vi "Main.vi"(0 "A":dbl=4.0 min=0.0, 5 "B":dbl=2.0, 7 "Calculate":bool, 11 "error in (no error)":errorcluster, 13 "Operation":T1) -> (4 "C":dbl=6.0, 15 "error out":errorcluster)   [LabVIEW 2021, in "Calculator.lvlib"]
doc: "This VI acts as a simple calculator using OOPS . There are four seperate child classes for each arithmetic operation which has its overriding method operation.vi . The user selects the operation to perform and gives the input. The output is displayed when calculate is pressed."
uses:
  Calculator.lvlib
  Controls/QueueOperations.ctl
  Controls/Operation.ctl
  Controls/DataCluster.ctl
  Classes/NumericOperation/NumericOperation.lvclass
  Classes/Child/Add/Add.lvclass
  Classes/Child/Subtract/Subtract.lvclass
  Classes/Child/Multiply/Multiply.lvclass
  Classes/Child/Divide/Divide.lvclass
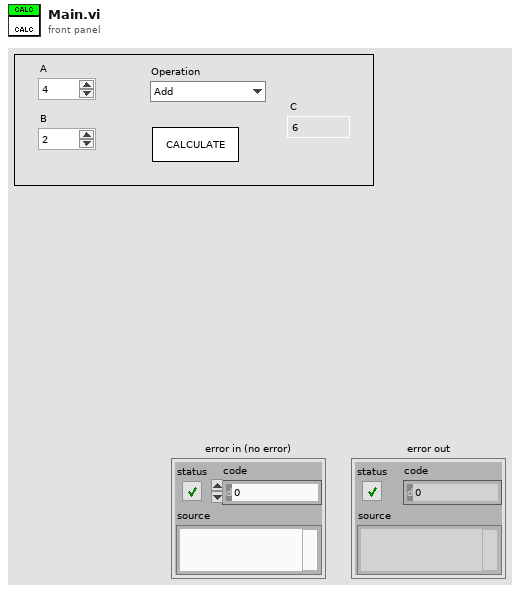
[diagram p1: front panel]
types:
  T1 = typedef "Calculator.lvlib/Operation.ctl" = enum16{"Add", "Subtract", "Multiply", "Divide"}
  T2 = typedef "Calculator.lvlib/QueueOperations.ctl" = enum16{"Create", "Enqueue", "EnqueueN", "Enqueue at Top", "Dequeue", "Flush", "Release"}
  T3 = typedef "Calculator.lvlib/DataCluster.ctl" = cluster{"A":dbl, "B":dbl, "C":dbl, "Operation":T1, "NumericOperation.lvclass":refnum<class "NumericOperation.lvclass">, "generic class reference":refnum<class "NumericOperation.lvclass">}
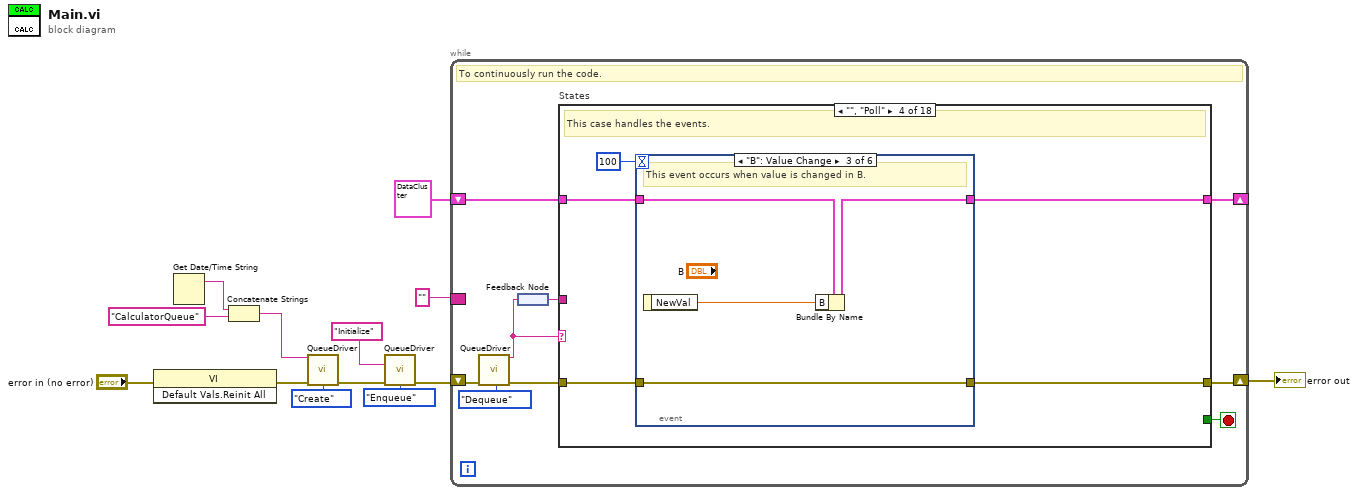
[diagram p0: block diagram]
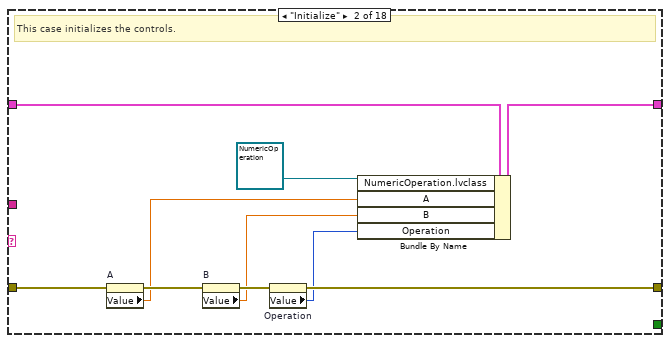
[diagram p3: hidden frame]
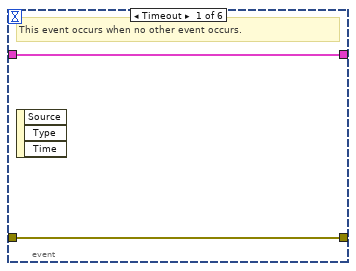
[diagram p5: hidden frame]
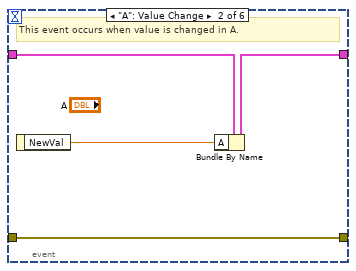
[diagram p6: hidden frame]
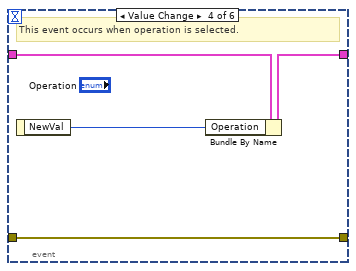
[diagram p7: hidden frame]
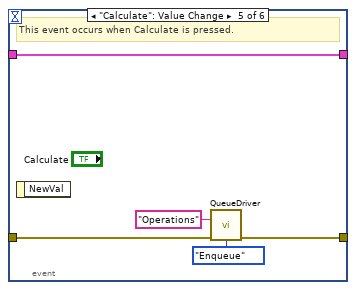
[diagram p8: hidden frame]
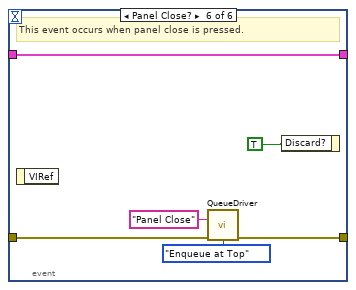
[diagram p9: hidden frame]
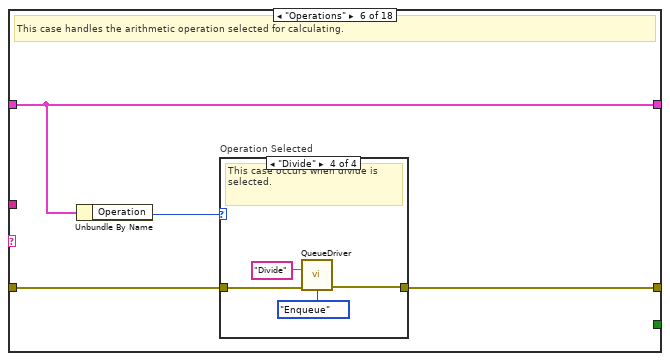
[diagram p11: hidden frame]
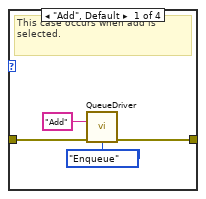
[diagram p12: hidden frame]
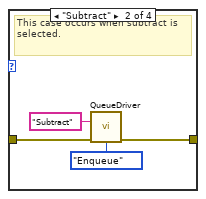
[diagram p13: hidden frame]
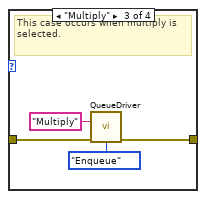
[diagram p14: hidden frame]
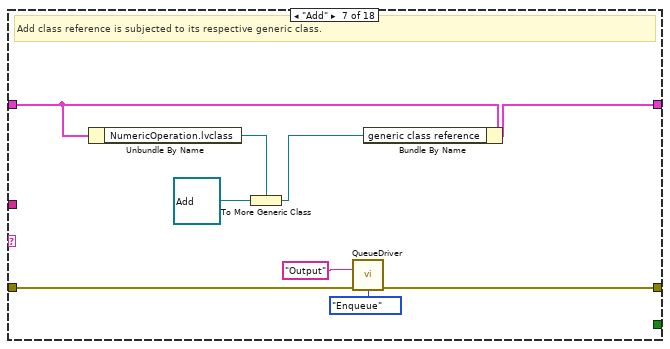
[diagram p15: hidden frame]
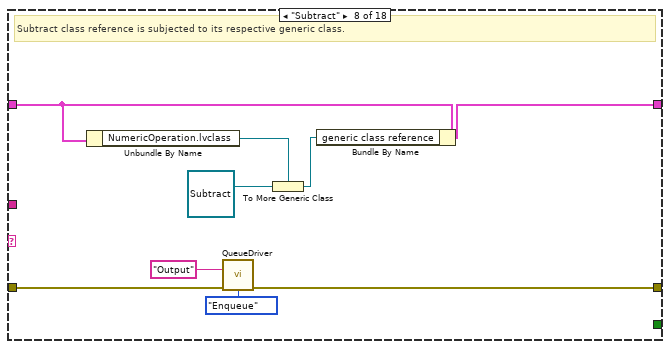
[diagram p16: hidden frame]
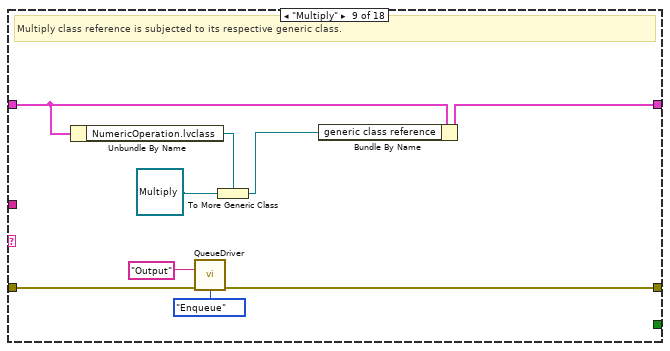
[diagram p17: hidden frame]
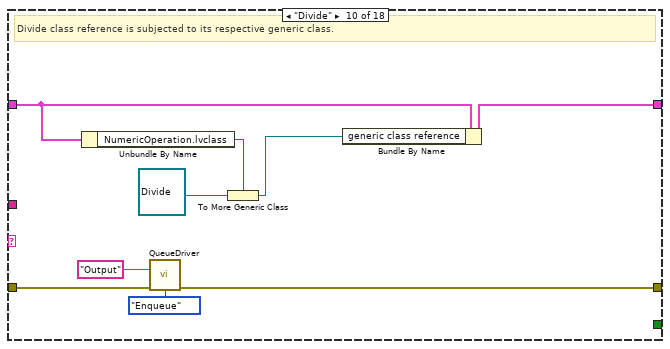
[diagram p18: hidden frame]
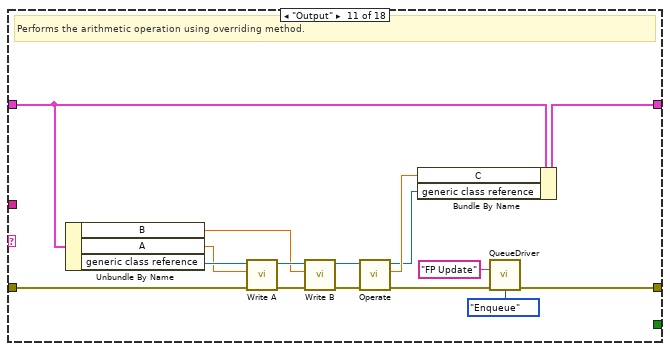
[diagram p19: hidden frame]
diagram:
  n1 = invoke class="VI" method="Default Vals.Reinit All"(error in="error in (no error)") -> (error out=w1:errorcluster)  [unwired: 2 in, 2 out]
  n2 = Get Date/Time String() -> (date string=w5:string)  [unwired: 3 in, 1 out]
  n3 = Concatenate Strings(w5, "CalculatorQueue" ("Queue Name")) -> (w3:string)
  n4 = call "QueueDriver.vi"("Queue Name"=w3, "error in (no error)"=w1, "Queue Operations"=QueueOperations."Create") -> ("error out"=w10:errorcluster)  [unwired: 11 in, 1 out]
  n5 = call "QueueDriver.vi"("State"="Initialize", "error in (no error)"=w10, "Queue Operations"=QueueOperations."Enqueue") -> ("error out"=w7:errorcluster)  [unwired: 11 in, 1 out]
  n6 = while {
    shift-right: [w20] -> _
    shift-left: T3 {"A"=0.0, "B"=0.0, "C"=0.0, "Operation"=enum."Add", "NumericOperation.lvclass"=refnum, "generic class reference"=refnum} -> [w21]
    shift-right: [w18] -> w12
    shift-left: w7 -> [w19]
    border: "" ("Dequeued Element") -> [_]
    stop <- w15 stop-if-true
    # "To continuously run the code."
    n7 = call "QueueDriver.vi"("error in (no error)"=w19, "Queue Operations"=QueueOperations."Dequeue") -> ("Dequeued Element"=w17:string, "error out"=w14:errorcluster)  [unwired: 12 in]
    n8 = feedback-in #1(w17) -> ()
    n9 = feedback #1() -> (w16:string)
    n10 = case "States" shown="\"\", \"Poll\"" w17 {
      tunnel: w21 -> [w24 w34 w36 w40 w68 w70 w94 w104 w112 w122 w140 w142 w144 w147 w150 w156 w161 w177]
      tunnel: [w24 w32 w36 w39 w68 w70 w93 w103 w111 w120 w138 w142 w144 w147 w150 w156 w161 w177] -> w20
      tunnel: [w23 w28 w35 w38 w67 w71 w92 w101 w110 w119 w136 w141 w143 w146 w151 w155 w163 w175] -> w18
      tunnel: w16 -> [_ _ _ _ _ _ _ _ _ _ _ _ _ _ _ _ w168 _]
      tunnel: [_ _ _ _ _ _ _ _ _ _ _ _ _ _ TRUE _ _ _] -> w15
      tunnel: w14 -> [w23 w31 w35 w37 w67 w69 w89 w98 w107 w116 w126 w141 w143 w146 w148 w155 w158 w175]
      frame "/******** Initialize********/" {
      }
      frame "Initialize" {
        # "This case initializes the controls."
        n11 = property on="A" class="DigNum (strict)"(error in=w31) -> (error out=w30:errorcluster, "Value"=w25:dbl)  [unwired: 1 in, 1 out]
        n12 = property on="B" class="DigNum (strict)"(error in=w30) -> (error out=w29:errorcluster, "Value"=w26:dbl)  [unwired: 1 in, 1 out]
        n13 = property on="Operation" class="Enum (strict)"(error in=w29) -> (error out=w28:errorcluster, "Value"=w27:T1)  [unwired: 1 in, 1 out]
        n14 = Bundle By Name(cluster=w34, "NumericOperation.lvclass"=refnum<class "NumericOperation.lvclass"> refnum, "A"=w25, "B"=w26, "Operation"=w27) -> (w32:T3)
      }
      frame "/******** Poll ********/" {
      }
      frame "", "Poll" {
        # "This case handles the events."
        n15 = event shown="[2] \"B\": Value Change" {
          selector: _ -> [_ _ _ _ _ _]
          dyn-events: _ -> [_ _ _ _ _ _]
          timeout: 100 -> [_ _ _ _ _ _]
          tunnel: w40 -> [w43 w47 w51 w55 w59 w63]
          tunnel: [w43 w45 w49 w53 w59 w63] -> w39
          tunnel: [w42 w44 w48 w52 w60 w65] -> w38
          tunnel: w37 -> [w42 w44 w48 w52 w56 w61]
          event Timeout {
            # "This event occurs when no other event occurs."
            n16 = event-data() -> ()  [unwired: 1 in, 3 out]
          }
          event "A": Value Change {
            # "This event occurs when value is changed in A."
            n17 = event-data() -> ("NewVal"=w46:dbl)  [unwired: 1 in]
            n18 = Bundle By Name(cluster=w47, "A"=w46) -> (w45:T3)
          }
          event "B": Value Change {
            # "This event occurs when value is changed in B."
            n19 = event-data() -> ("NewVal"=w50:dbl)  [unwired: 1 in]
            n20 = Bundle By Name(cluster=w51, "B"=w50) -> (w49:T3)
          }
          event Value Change {
            # "This event occurs when operation is selected."
            n21 = event-data() -> ("NewVal"=w54:T1)  [unwired: 1 in]
            n22 = Bundle By Name(cluster=w55, "Operation"=w54) -> (w53:T3)
          }
          event "Calculate": Value Change {
            # "This event occurs when Calculate is pressed."
            n23 = event-data() -> ()  [unwired: 1 in, 1 out]
            n24 = call "QueueDriver.vi"("State"="Operations", "error in (no error)"=w56, "Queue Operations"=QueueOperations."Enqueue") -> ("error out"=w60:errorcluster)  [unwired: 11 in, 1 out]
          }
          event Panel Close? {
            # "This event occurs when panel close is pressed."
            n25 = event-data() -> ()  [unwired: 1 in, 1 out]
            n26 = call "QueueDriver.vi"("State"="Panel Close", "error in (no error)"=w61, "Queue Operations"=QueueOperations."Enqueue at Top") -> ("error out"=w65:errorcluster)  [unwired: 11 in, 1 out]
            n27 = event-data("Discard?"=TRUE) -> ()  [unwired: 1 in, 1 out]
          }
        }
      }
      frame "/******** Functionalities ********/" {
      }
      frame "Operations" {
        # "This case handles the arithmetic operation selected for calculating."
        n28 = Unbundle By Name(w70) -> ("Operation"=w72:T1)
        n29 = case "Operation Selected" shown="\"Divide\"" w72 {
          tunnel: [w76 w80 w84 w88] -> w71
          tunnel: w69 -> [w73 w77 w81 w85]
          frame "Add", Default {
            # "This case occurs when add is selected."
            n30 = call "QueueDriver.vi"("State"="Add", "error in (no error)"=w73, "Queue Operations"=QueueOperations."Enqueue") -> ("error out"=w76:errorcluster)  [unwired: 11 in, 1 out]
          }
          frame "Subtract" {
            # "This case occurs when subtract is selected."
            n31 = call "QueueDriver.vi"("State"="Subtract", "error in (no error)"=w77, "Queue Operations"=QueueOperations."Enqueue") -> ("error out"=w80:errorcluster)  [unwired: 11 in, 1 out]
          }
          frame "Multiply" {
            # "This case occurs when multiply is selected."
            n32 = call "QueueDriver.vi"("State"="Multiply", "error in (no error)"=w81, "Queue Operations"=QueueOperations."Enqueue") -> ("error out"=w84:errorcluster)  [unwired: 11 in, 1 out]
          }
          frame "Divide" {
            # "This case occurs when divide is selected."
            n33 = call "QueueDriver.vi"("State"="Divide", "error in (no error)"=w85, "Queue Operations"=QueueOperations."Enqueue") -> ("error out"=w88:errorcluster)  [unwired: 11 in, 1 out]
          }
        }
      }
      frame "Add" {
        # "Add class reference is subjected to its respective generic class."
        n34 = Unbundle By Name(w94) -> ("NumericOperation.lvclass"=w97:refnum<class "NumericOperation.lvclass">)
        n35 = To More Generic Class(target class=w97, reference=refnum<class "Add.lvclass"> refnum ("Add.lvclass")) -> (generic class reference=w95:refnum<class "NumericOperation.lvclass">)
        n36 = call "QueueDriver.vi"("State"="Output", "error in (no error)"=w89, "Queue Operations"=QueueOperations."Enqueue") -> ("error out"=w92:errorcluster)  [unwired: 11 in, 1 out]
        n37 = Bundle By Name(cluster=w94, "generic class reference"=w95) -> (w93:T3)
      }
      frame "Subtract" {
        # "Subtract class reference is subjected to its respective generic class."
        n38 = Unbundle By Name(w104) -> ("NumericOperation.lvclass"=w106:refnum<class "NumericOperation.lvclass">)
        n39 = call "QueueDriver.vi"("State"="Output", "error in (no error)"=w98, "Queue Operations"=QueueOperations."Enqueue") -> ("error out"=w101:errorcluster)  [unwired: 11 in, 1 out]
        n40 = To More Generic Class(target class=w106, reference=refnum<class "Subtract.lvclass"> refnum ("Subtract.lvclass")) -> (generic class reference=w102:refnum<class "NumericOperation.lvclass">)
        n41 = Bundle By Name(cluster=w104, "generic class reference"=w102) -> (w103:T3)
      }
      frame "Multiply" {
        # "Multiply class reference is subjected to its respective generic class."
        n42 = Unbundle By Name(w112) -> ("NumericOperation.lvclass"=w114:refnum<class "NumericOperation.lvclass">)
        n43 = call "QueueDriver.vi"("State"="Output", "error in (no error)"=w107, "Queue Operations"=QueueOperations."Enqueue") -> ("error out"=w110:errorcluster)  [unwired: 11 in, 1 out]
        n44 = To More Generic Class(target class=w114, reference=refnum<class "Multiply.lvclass"> refnum ("Multiply.lvclass")) -> (generic class reference=w113:refnum<class "NumericOperation.lvclass">)
        n45 = Bundle By Name(cluster=w112, "generic class reference"=w113) -> (w111:T3)
      }
      frame "Divide" {
        # "Divide class reference is subjected to its respective generic class."
        n46 = Unbundle By Name(w122) -> ("NumericOperation.lvclass"=w124:refnum<class "NumericOperation.lvclass">)
        n47 = call "QueueDriver.vi"("State"="Output", "error in (no error)"=w116, "Queue Operations"=QueueOperations."Enqueue") -> ("error out"=w119:errorcluster)  [unwired: 11 in, 1 out]
        n48 = To More Generic Class(target class=w124, reference=refnum<class "Divide.lvclass"> refnum ("Divide.lvclass")) -> (generic class reference=w121:refnum<class "NumericOperation.lvclass">)
        n49 = Bundle By Name(cluster=w122, "generic class reference"=w121) -> (w120:T3)
      }
      frame "Output" {
        # "Performs the arithmetic operation using overriding method."
        n50 = Unbundle By Name(w140) -> ("B"=w127:dbl, "A"=w128:dbl, "generic class reference"=w131:refnum<class "NumericOperation.lvclass">)
        n51 = call-dynamic "Write A.vi"("error in (no error)"=w126, "A"=w128, "NumericOperation in"=w131) -> ("error out"=w133:errorcluster, "NumericOperation out"=w130:refnum<class "NumericOperation.lvclass">)  [unwired: 7 in]
        n52 = call-dynamic "Write B.vi"("error in (no error)"=w133, "B"=w127, "NumericOperation in"=w130) -> ("error out"=w132:errorcluster, "NumericOperation out"=w129:refnum<class "NumericOperation.lvclass">)  [unwired: 7 in]
        n53 = call-dynamic "Operate.vi"("error in (no error)"=w132, "NumericOperation in"=w129) -> ("error out"=w137:errorcluster, "C"=w139:dbl, "NumericOperation out"=w125:refnum<class "NumericOperation.lvclass">)  [unwired: 7 in]
        n54 = Bundle By Name(cluster=w140, "C"=w139, "generic class reference"=w125) -> (w138:T3)
        n55 = call "QueueDriver.vi"("State"="FP Update", "error in (no error)"=w137, "Queue Operations"=QueueOperations."Enqueue") -> ("error out"=w136:errorcluster)  [unwired: 11 in, 1 out]
      }
      frame "/******** Front Panel Updates ********/" {
      }
      frame "FP Update" {
        # "Updates the front panel indicators."
        n56 = Unbundle By Name(w144) -> ("C"=→"C":dbl)
      }
      frame "/******** Panel Close ********/" {
      }
      frame "Panel Close" {
        # "Stops the running VI ."
        n57 = call "QueueDriver.vi"("error in (no error)"=w148, "Queue Operations"=QueueOperations."Flush") -> ("error out"=w152:errorcluster)  [unwired: 12 in, 1 out]
        n58 = call "QueueDriver.vi"("error in (no error)"=w152, "Queue Operations"=QueueOperations."Release") -> ("error out"=w151:errorcluster)  [unwired: 12 in, 1 out]
      }
      frame "/******** Error handling ********/" {
      }
      frame "Error" {
        # "This case handles the error."
        n59 = Unbundle By Name(w158) -> ("code"=w159:i32, "source"=w157:string)
        n60 = call <vilib>:"Clear Errors.vi"("error in (no error)"=w158) -> ("error out"=w160:errorcluster)  [unwired: 5 in, 1 out]
        n61 = Format Into String(format string="Error occurred in state \"%s\"!!\nError Code: %d\nError Source: %s\n\nDo you wish to continue?", error in=w160, w168, w159, w157) -> (resulting string=w165:string, error out=w164:errorcluster)  [unwired: 1 in]
        n62 = Two Button Dialog(message=w165, 1:"Exit" ("F button name (\"Cancel\")"), 2:"Continue" ("T button name (\"OK\")")) -> (T button?=w162:bool)
        n63 = case "Continue?" shown="False" w162 {
          tunnel: w164 -> [w173 w174]
          tunnel: [w172 w174] -> w163
          frame False {
            n64 = call "QueueDriver.vi"("State"="Panel Close", "error in (no error)"=w173, "Queue Operations"=QueueOperations."Enqueue at Top") -> ("error out"=w172:errorcluster)  [unwired: 11 in, 1 out]
          }
          frame True {
          }
        }
      }
      frame Default {
        # "This case handles the developer error."
        n65 = One Button Dialog(message="Developer error occured!!") -> ()  [unwired: 1 in, 1 out]
      }
    }
  }
  "error out" <- w12
